vi "DecryptEndpointPasswords.vi"(8 "error in (no error)":errorcluster, 10 "srp":T2, 11 "EncryptedEndpointPasswords":T1) -> (0 "error out":errorcluster, 2 "new password list":string, 3 "wireless endpoint auths":string)   [LabVIEW 2017, in "ServerComm.lvlib"]
uses:
  <vilib>/addons/InsightCM/Devices/Shared/Common/ServerComm/ServerComm.lvlib
  <vilib>/addons/InsightCM/SRP/controls/DVR_data.ctl
  <vilib>/addons/InsightCM/SRP/controls/data.ctl
  <vilib>/addons/InsightCM/MessageBus/Base/controls/EncryptedEndpointPasswords.ctl
  <vilib>/addons/InsightCM/SRP/SRP.lvlib
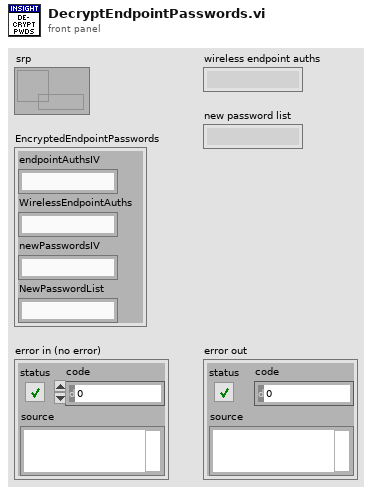
[diagram p1: front panel]
types:
  T1 = typedef "EncryptedEndpointPasswords.ctl" = cluster{"endpointAuthsIV":string, "WirelessEndpointAuths":string, "newPasswordsIV":string, "NewPasswordList":string}
  T2 = typedef "SRP.lvlib/DVR_data.ctl" = refnum<data-value>
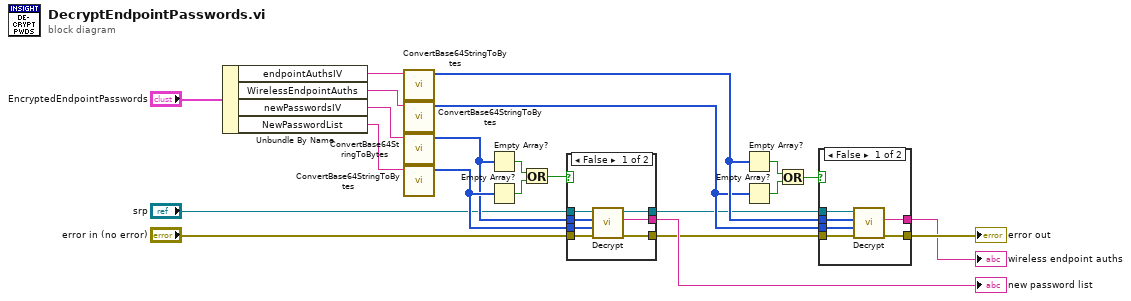
[diagram p0: block diagram]
diagram:
  n1 = Unbundle By Name("EncryptedEndpointPasswords") -> ("endpointAuthsIV"=w3:string, "WirelessEndpointAuths"=w4:string, "newPasswordsIV"=w5:string, "NewPasswordList"=w6:string)
  n2 = call <vilib>:"ConvertBase64StringToBytes.vi"("Base64 string"=w3) -> ("U8 array"=w20:u8[])  [unwired: 9 in, 1 out]
  n3 = call <vilib>:"ConvertBase64StringToBytes.vi"("Base64 string"=w4) -> ("U8 array"=w19:u8[])  [unwired: 9 in, 1 out]
  n4 = call <vilib>:"ConvertBase64StringToBytes.vi"("Base64 string"=w5) -> ("U8 array"=w11:u8[])  [unwired: 9 in, 1 out]
  n5 = call <vilib>:"ConvertBase64StringToBytes.vi"("Base64 string"=w6) -> ("U8 array"=w12:u8[])  [unwired: 9 in, 1 out]
  n6 = Empty Array?(array=w11) -> (empty?=w15:bool)
  n7 = Empty Array?(array=w12) -> (empty?=w16:bool)
  n8 = Or(x=w15, y=w16) -> (x .or. y?=w14:bool)
  n9 = case shown="False" w14 {
    tunnel: "error in (no error)" -> [w23 w30]
    tunnel: "srp" -> [w29 w31]
    tunnel: w11 -> [w28 _]
    tunnel: w12 -> [w27 _]
    tunnel: [w26 w31] -> w7
    tunnel: [w25 w30] -> w8
    tunnel: [w24 _] -> w9
    frame False {
      n10 = call <vilib>:"Decrypt.vi"("error in (no error)"=w23, "Configuration"=w27, "IV"=w28, "srp"=w29) -> ("error out"=w25:errorcluster, "output"=w24:string, "srp"=w26:T2)  [unwired: 5 in]
    }
    frame True {
    }
  }
  "new password list" <- w9
  n11 = Empty Array?(array=w20) -> (empty?=w18:bool)
  n12 = Empty Array?(array=w19) -> (empty?=w17:bool)
  n13 = Or(x=w18, y=w17) -> (x .or. y?=w21:bool)
  n14 = case shown="False" w21 {
    tunnel: w7 -> [w37 _]
    tunnel: w8 -> [w36 w38]
    tunnel: w20 -> [w35 _]
    tunnel: w19 -> [w34 _]
    tunnel: [w33 _] -> w10
    tunnel: [w32 w38] -> w22
    frame False {
      n15 = call <vilib>:"Decrypt.vi"("error in (no error)"=w36, "Configuration"=w34, "IV"=w35, "srp"=w37) -> ("error out"=w32:errorcluster, "output"=w33:string)  [unwired: 5 in, 1 out]
    }
    frame True {
    }
  }
  "error out" <- w22
  "wireless endpoint auths" <- w10
